vi "Do.vi"(8 "error in (no error)":errorcluster, 10 "Actor in":refnum<class "Actor.lvclass">, 11 "Change Heater SP MSG":refnum<class "Change Heater SP MSG.lvclass">) -> (0 "error out":errorcluster, 2 "Actor out":refnum<class "Actor.lvclass">)   [LabVIEW 2017, in "Controller.lvlib" / "Change Heater SP MSG.lvclass"]
doc: "(<B>Filename</B>: Actor Framework.lvlib:Message.lvclass:Do.vi)\n\nDefines what a message does when it is received by an actor. Generally, a message instructs an actor to invoke one of its methods. By default, this method does nothing. A child class must override it to define behavior. Create a child class by using the Actor Framework Message Maker dialog box."
uses:
  Change Heater SP MSG.lvclass
  <vilib>/ActorFramework/Actor/Actor.lvclass
  Change Heater SP MSG.lvclass/Change Heater SP MSG.ctl
  gController.lvclass
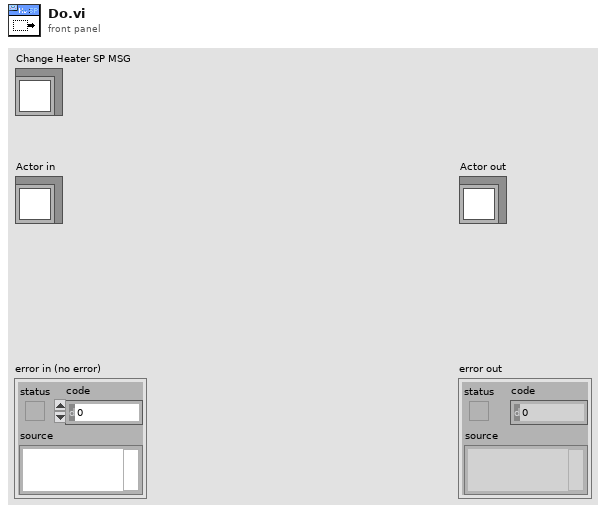
[diagram p1: front panel]
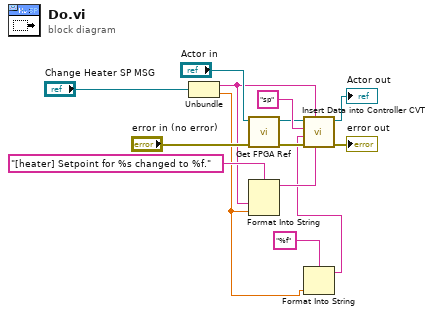
[diagram p0: block diagram]
diagram:
  n1 = Unbundle("Change Heater SP MSG") -> (w5:string, w2:dbl)
  n2 = call "Get FPGA Ref.vi"("error in (no error)"="error in (no error)", "Actor In"="Actor in") -> ("error out"=w8:errorcluster, "Actor Out"=w11:refnum<class "Actor.lvclass">)  [unwired: 7 in, 1 out]
  n3 = Format Into String(format string="[heater] Setpoint for %s changed to %f.", w5, w2) -> (resulting string=w4:string)  [unwired: 2 in, 1 out]
  n4 = Format Into String(format string="%f", w2) -> (resulting string=w1:string)  [unwired: 2 in, 1 out]
  n5 = call "Insert Data into Controller CVT.vi"("Update MSG"=w4, "Group"=w5, "error in"=w8, "Data"=w1, "tag"="sp", "Actor in"=w11) -> ("error out"=→"error out":errorcluster, "Actor Out"=→"Actor out":refnum<class "Actor.lvclass">)  [unwired: 4 in]
